vi "Read Digital Voltmeter Statistics.vi"(8 "error in (no error)":errorcluster, 11 "VISA resource name":refnum<visa-resource-name>) -> (0 "error out":errorcluster, 1 "Minimum Value":dbl, 2 "Maximum Value":dbl, 3 "VISA resource name out":refnum<visa-resource-name>)   [LabVIEW 2017, in "Scope.lvlib" / "Tektronix DPO MSO 2000 4000 Series.lvlib"]
doc: "Reads the maximum and minimum Digital Voltmeter readout value over the entire time that the Digital Voltmeter has been on since the last change using <B>Configure Digital Voltmeter</B> VI or <B>Reset Digital Voltmeter</B> VI.\n\n<B>Notes:</B>\n(1) This VI is available for MDO3000 Series only.\n\n(2) Requires option MDO3DVM to be installed."
uses:
  Tektronix DPO MSO 2000 4000 Series.lvlib
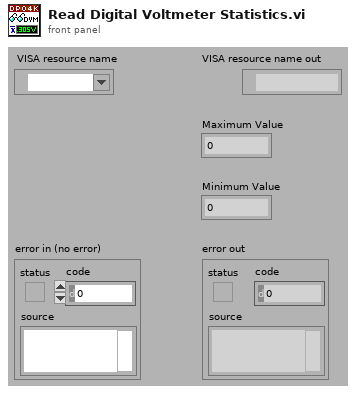
[diagram p1: front panel]
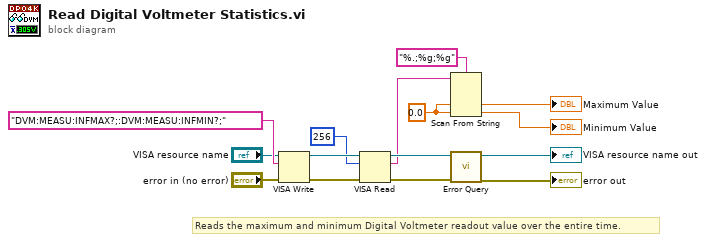
[diagram p0: block diagram]
diagram:
  w9 = 0.0 ("default value 1")
  # "Reads the maximum and minimum Digital Voltmeter readout value over the entire time."
  n1 = VISA Write(VISA resource name="VISA resource name", write buffer="DVM:MEASU:INFMAX?;:DVM:MEASU:INFMIN?;", error in (no error)="error in (no error)") -> (VISA resource name out=w8:refnum<visa-resource-name>, error out=w7:errorcluster)  [unwired: 1 out]
  n2 = VISA Read(VISA resource name=w8, byte count=u32 256, error in (no error)=w7) -> (VISA resource name out=w6:refnum<visa-resource-name>, read buffer=w4:string, error out=w5:errorcluster)  [unwired: 1 out]
  n3 = Scan From String(format string="%.;%g;%g", input string=w4, default 1=w9, default 2=w9) -> (output 1=→"Maximum Value":dbl, output 2=→"Minimum Value":dbl)  [unwired: 2 in, 3 out]
  n4 = call "Error Query.vi"("error in (no error)"=w5, "VISA resource name"=w6) -> ("error out"=→"error out":errorcluster, "VISA resource name out"=→"VISA resource name out":refnum<visa-resource-name>)  [unwired: 6 in, 2 out]
